vi "Saw Wave Generator.vi"(0 "frequency (periods/tick)":fxp<+,32,0>=0.0002500000409781933, 1 "reset":bool, 5 "phase offset (periods)":fxp<+,32,0>) -> (4 "saw out":i16)   [LabVIEW 2015]
doc: "Generates a point-by-point triangle wave using direct digital synthesis. The synthesis runs continuously from the top-level FPGA target clock to produce an accurate real-time frequency. Each execution of this VI returns the most recent sample produced by the underlying synthesis engine."
uses:
  <vilib>/rvi/Analysis/common/FxpNativeNode/niFpgaFxpNative.xnode
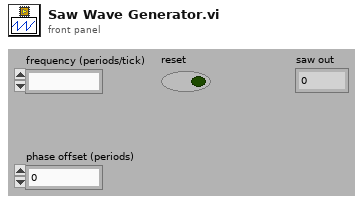
[diagram p1: front panel]
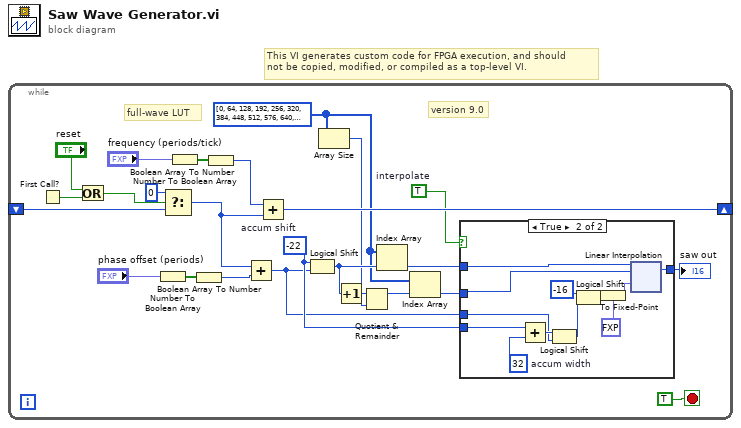
[diagram p0: block diagram]
diagram:
  # "This VI generates custom code for FPGA execution, and should\nnot be copied, modified, or compiled as a top-level VI."
  n1 = while {
    shift-right: [w24] -> _
    shift-left: _ -> [w17]
    stop <- TRUE stop-if-true
    w1 = i16[] [0, 64, 128, 192, 256, 320, 384, 448, 512, 576, 640, 704, 768, 832, 896, 960, 1024, 1088, 1152, 1216, 1280, 1344, 1408, 1472, 1536, 1600, 1664, 1728, 1792, 1856, 1920, 1984, 2048, 2112, 2176, 2240, 2304, 2368, 2432, 2496, 2560, 2624, 2688, 2752, 2816, 2880, 2944, 3008, 3072, 3136, 3200, 3264, 3328, 3392, 3456, 3520, 3584, 3648, 3712, 3776, 3840, 3904, 3968, 4032, 4096, 4160, 4224, 4288, 4352, 4416, 4480, 4544, 4608, 4672, 4736, 4800, 4864, 4928, 4992, 5056, 5120, 5184, 5248, 5312, 5376, 5440, 5504, 5568, 5632, 5696, 5760, 5824, 5888, 5952, 6016, 6080, 6144, 6208, 6272, 6336, 6400, 6464, 6528, 6592, 6656, 6720, 6784, 6848, 6912, 6976, 7040, 7104, 7168, 7232, 7296, 7360, 7424, 7488, 7552, 7616, 7680, 7744, 7808, 7872, 7936, 8000, 8064, 8128, 8192, 8256, 8320, 8384, 8448, 8512, 8576, 8640, 8704, 8768, 8832, 8896, 8960, 9024, 9088, 9152, 9216, 9280, 9344, 9408, 9472, 9536, 9600, 9664, 9728, 9792, 9856, 9920, 9984, 10048, 10112, 10176, 10240, 10304, 10368, 10432, 10496, 10560, 10624, 10688, 10752, 10816, 10880, 10944, 11008, 11072, 11136, 11200, 11264, 11328, 11392, 11456, 11520, 11584, 11648, 11712, 11776, 11840, 11904, 11968, 12032, 12096, 12160, 12224, 12288, 12352, 12416, 12480, 12544, 12608, 12672, 12736, 12800, 12864, 12928, 12992, 13056, 13120, 13184, 13248, 13312, 13376, 13440, 13504, 13568, 13632, 13696, 13760, 13824, 13888, 13952, 14016, 14080, 14144, 14208, 14272, 14336, 14400, 14464, 14528, 14592, 14656, 14720, 14784, 14848, 14912, 14976, 15040, 15104, 15168, 15232, 15296, 15360, 15424, 15488, 15552, 15616, 15680, 15744, 15808, 15872, 15936, 16000, 16063, 16127, 16191, 16255, 16319, 16383, 16447, 16511, 16575, 16639, 16703, 16767, 16831, 16895, 16959, 17023, 17087, 17151, 17215, 17279, 17343, 17407, 17471, 17535, 17599, 17663, 17727, 17791, 17855, 17919, 17983, 18047, 18111, 18175, 18239, 18303, 18367, 18431, 18495, 18559, 18623, 18687, 18751, 18815, 18879, 18943, 19007, 19071, 19135, 19199, 19263, 19327, 19391, 19455, 19519, 19583, 19647, 19711, 19775, 19839, 19903, 19967, 20031, 20095, 20159, 20223, 20287, 20351, 20415, 20479, 20543, 20607, 20671, 20735, 20799, 20863, 20927, 20991, 21055, 21119, 21183, 21247, 21311, 21375, 21439, 21503, 21567, 21631, 21695, 21759, 21823, 21887, 21951, 22015, 22079, 22143, 22207, 22271, 22335, 22399, 22463, 22527, 22591, 22655, 22719, 22783, 22847, 22911, 22975, 23039, 23103, 23167, 23231, 23295, 23359, 23423, 23487, 23551, 23615, 23679, 23743, 23807, 23871, 23935, 23999, 24063, 24127, 24191, 24255, 24319, 24383, 24447, 24511, 24575, 24639, 24703, 24767, 24831, 24895, 24959, 25023, 25087, 25151, 25215, 25279, 25343, 25407, 25471, 25535, 25599, 25663, 25727, 25791, 25855, 25919, 25983, 26047, 26111, 26175, 26239, 26303, 26367, 26431, 26495, 26559, 26623, 26687, 26751, 26815, 26879, 26943, 27007, 27071, 27135, 27199, 27263, 27327, 27391, 27455, 27519, 27583, 27647, 27711, 27775, 27839, 27903, 27967, 28031, 28095, 28159, 28223, 28287, 28351, 28415, 28479, 28543, 28607, 28671, 28735, 28799, 28863, 28927, 28991, 29055, 29119, 29183, 29247, 29311, 29375, 29439, 29503, 29567, 29631, 29695, 29759, 29823, 29887, 29951, 30015, 30079, 30143, 30207, 30271, 30335, 30399, 30463, 30527, 30591, 30655, 30719, 30783, 30847, 30911, 30975, 31039, 31103, 31167, 31231, 31295, 31359, 31423, 31487, 31551, 31615, 31679, 31743, 31807, 31871, 31935, 31999, 32063, 32127, 32191, 32255, 32319, 32383, 32447, 32511, 32575, 32639, 32703, 32767, -32768, -32704, -32639, -32575, -32511, -32447, -32382, -32318, -32254, -32190, -32125, -32061, -31997, -31933, -31868, -31804, -31740, -31676, -31611, -31547, -31483, -31419, -31354, -31290, -31226, -31162, -31097, -31033, -30969, -30905, -30840, -30776, -30712, -30648, -30583, -30519, -30455, -30391, -30326, -30262, -30198, -30134, -30069, -30005, -29941, -29877, -29812, -29748, -29684, -29620, -29555, -29491, -29427, -29363, -29298, -29234, -29170, -29106, -29041, -28977, -28913, -28849, -28784, -28720, -28656, -28592, -28527, -28463, -28399, -28335, -28270, -28206, -28142, -28078, -28013, -27949, -27885, -27821, -27756, -27692, -27628, -27564, -27499, -27435, -27371, -27307, -27242, -27178, -27114, -27050, -26985, -26921, -26857, -26793, -26728, -26664, -26600, -26536, -26471, -26407, -26343, -26279, -26214, -26150, -26086, -26022, -25957, -25893, -25829, -25765, -25700, -25636, -25572, -25508, -25443, -25379, -25315, -25251, -25186, -25122, -25058, -24994, -24929, -24865, -24801, -24737, -24672, -24608, -24544, -24480, -24415, -24351, -24287, -24223, -24158, -24094, -24030, -23966, -23901, -23837, -23773, -23709, -23644, -23580, -23516, -23452, -23387, -23323, -23259, -23195, -23130, -23066, -23002, -22938, -22873, -22809, -22745, -22681, -22616, -22552, -22488, -22424, -22359, -22295, -22231, -22167, -22102, -22038, -21974, -21910, -21845, -21781, -21717, -21653, -21588, -21524, -21460, -21396, -21331, -21267, -21203, -21139, -21074, -21010, -20946, -20882, -20817, -20753, -20689, -20625, -20560, -20496, -20432, -20368, -20303, -20239, -20175, -20111, -20046, -19982, -19918, -19854, -19789, -19725, -19661, -19597, -19532, -19468, -19404, -19340, -19275, -19211, -19147, -19083, -19018, -18954, -18890, -18826, -18761, -18697, -18633, -18569, -18504, -18440, -18376, -18312, -18247, -18183, -18119, -18055, -17990, -17926, -17862, -17798, -17733, -17669, -17605, -17541, -17476, -17412, -17348, -17284, -17219, -17155, -17091, -17027, -16962, -16898, -16834, -16770, -16705, -16641, -16577, -16512, -16448, -16384, -16320, -16255, -16191, -16127, -16063, -15998, -15934, -15870, -15806, -15741, -15677, -15613, -15549, -15484, -15420, -15356, -15292, -15227, -15163, -15099, -15035, -14970, -14906, -14842, -14778, -14713, -14649, -14585, -14521, -14456, -14392, -14328, -14264, -14199, -14135, -14071, -14007, -13942, -13878, -13814, -13750, -13685, -13621, -13557, -13493, -13428, -13364, -13300, -13236, -13171, -13107, -13043, -12979, -12914, -12850, -12786, -12722, -12657, -12593, -12529, -12465, -12400, -12336, -12272, -12208, -12143, -12079, -12015, -11951, -11886, -11822, -11758, -11694, -11629, -11565, -11501, -11437, -11372, -11308, -11244, -11180, -11115, -11051, -10987, -10923, -10858, -10794, -10730, -10666, -10601, -10537, -10473, -10409, -10344, -10280, -10216, -10152, -10087, -10023, -9959, -9895, -9830, -9766, -9702, -9638, -9573, -9509, -9445, -9381, -9316, -9252, -9188, -9124, -9059, -8995, -8931, -8867, -8802, -8738, -8674, -8610, -8545, -8481, -8417, -8353, -8288, -8224, -8160, -8096, -8031, -7967, -7903, -7839, -7774, -7710, -7646, -7582, -7517, -7453, -7389, -7325, -7260, -7196, -7132, -7068, -7003, -6939, -6875, -6811, -6746, -6682, -6618, -6554, -6489, -6425, -6361, -6297, -6232, -6168, -6104, -6040, -5975, -5911, -5847, -5783, -5718, -5654, -5590, -5526, -5461, -5397, -5333, -5269, -5204, -5140, -5076, -5012, -4947, -4883, -4819, -4755, -4690, -4626, -4562, -4498, -4433, -4369, -4305, -4241, -4176, -4112, -4048, -3984, -3919, -3855, -3791, -3727, -3662, -3598, -3534, -3470, -3405, -3341, -3277, -3213, -3148, -3084, -3020, -2956, -2891, -2827, -2763, -2699, -2634, -2570, -2506, -2442, -2377, -2313, -2249, -2185, -2120, -2056, -1992, -1928, -1863, -1799, -1735, -1671, -1606, -1542, -1478, -1414, -1349, -1285, -1221, -1157, -1092, -1028, -964, -900, -835, -771, -707, -642, -578, -514, -450, -385, -321, -257, -193, -128, -64, 0] ("Array 2")
    w20 = TRUE  # interpolate
    w19 = i8 -22  # accum shift
    # "version 9.0"
    # "full-wave LUT"
    n2 = First Call?() -> (First Call?: T/F=w15:bool)
    n3 = Or(x="reset", y=w15) -> (x .or. y?=w14:bool)
    n4 = Number To Boolean Array(number="phase offset (periods)") -> (Boolean array=w4:bool[])
    n5 = Select(t=u32 0, s=w14, f=w17) -> (s? t:f=w22:u32)
    n6 = Number To Boolean Array(number="frequency (periods/tick)") -> (Boolean array=w7:bool[])
    n7 = Boolean Array To Number(Boolean array=w4) -> (number=w2:u32)
    n8 = Boolean Array To Number(Boolean array=w7) -> (number=w5:u32)
    n9 = Add(x=w22, y=w2) -> (x+y=w18:u32)
    n10 = Add(x=w5, y=w22) -> (x+y=w24:u32)
    n11 = Logical Shift(y=w19, x=w18) -> (x << y=w12:u32)
    n12 = Array Size(array=w1) -> (size(s)=w8:i32)
    n13 = Increment(x=w12) -> (x+1=w13:u32)
    n14 = Quotient & Remainder(x=w13, y=w8) -> (x-y*floor(x/y)=w10:u32)  [unwired: 1 out]
    n15 = Index Array(array=w1, index=w12) -> (element=w11:i16)
    n16 = Index Array(array=w1, index=w10) -> (element=w9:i16)
    n17 = case shown="True" w20 {
      tunnel: w11 -> [w26 w29]
      tunnel: [w26 w28] -> w21
      tunnel: w19 -> [_ w38]
      tunnel: w18 -> [_ w35]
      tunnel: w9 -> [_ w30]
      frame False {
      }
      frame True {
        w37 = i8 32  # accum width
        n18 = Add(x=w38, y=w37) -> (x+y=w36:i8)
        n19 = Logical Shift(y=w36, x=w35) -> (x << y=w34:u32)
        n20 = Logical Shift(y=-16, x=w34) -> (x << y=w32:u32)
        n21 = To Fixed-Point(fixed-point type=fxp<+,16,0> 0.0, number=w32) -> (fixed-point=w31:fxp<+,16,0>)
        n22 = xnode ("Linear Interpolation")("y0"=w29, "y1"=w30, "x"=w31) -> ("y"=w28:i16)
      }
    }
    "saw out" <- w21
  }
